vi "PCO_SetRecorderSubmode.vi"(8 "error in (no error)":errorcluster {"code" format="%x"}, 10 "wRecSubmode":u16(ring) items=["sequence", "ring buffer"], 11 "ph":u64) -> (0 "error out":errorcluster {"code" format="%x"}, 2 "ErrorMessage":i32 format="%x", 3 "ph out":u64)   [LabVIEW 2019, in "SDK.lvlib" / "RecordingControl.lvlib"]
doc: "<b>Description:</b>\nThis function sets the recorder submode of the camera. Recorder submode is only available if PCO_SetStorageMode is set to [recorder].\nRecorder submode can be set to [sequence] or [ring buffer].\n\n<b>-->RecorderSubmode: [sequence]</b>\nRecording is stopped, when the last buffer in the segment is reached\nNo images are overwritten\nRecording can be stopped by software\n\n<b>-->RecorderSubmode: [ring buffer]</b>\nCamera records continuously into ring buffer\nThe oldest images are overwritten, if a buffer overflows occures due to long recording times\nRecording must be stopped by software or with an stop event\n\n<b>Supported camera type:</b>\npco.dimax, pco.pixelfly usb, pco.ultraviolet, pco.1200, pco.1300, pco.1400, pco.1600, pco.2000, pco.4000\n\n<b>Descriptor dependency:</b>\ndwGeneralCapsDESC1: NO_RECORDER"
uses:
  RecordingControl.lvlib
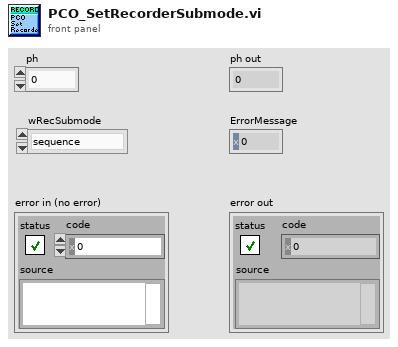
[diagram p1: front panel]
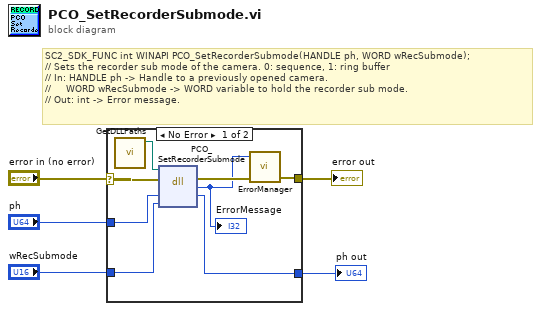
[diagram p0: block diagram]
diagram:
  # "SC2_SDK_FUNC int WINAPI PCO_SetRecorderSubmode(HANDLE ph, WORD wRecSubmode);\n// Sets the recorder sub mode of the camera. 0: sequence, 1: ring buffer\n// In: HANDLE ph -> Handle to a previously opened camera.\n//     WORD wRecSubmode -> WORD variable to hold the recorder sub mode.\n// Out: int -> Error message."
  n1 = case shown="No Error" "error in (no error)" {
    selector: "error in (no error)" -> [w10 w15]
    tunnel: "ph" -> [w13 w14]
    tunnel: [w12 w14] -> w4
    tunnel: "wRecSubmode" -> [w11 _]
    tunnel: [w8 w15] -> w2
    frame No Error {
      n2 = call "GetDLLPaths.vi"() -> ("SC2_Cam_Path"=w6:path)  [unwired: 9 in, 2 out]
      n3 = dll-call lib="?" fn="PCO_SetRecorderSubmode"(path in=w6, error in=w10, "ph"=w13, "wRecSubmode"=w11) -> (error out=w9:errorcluster, "return type"=w7:i32, "ph"=w12:u64)  [unwired: 2 in, 1 out]
      "ErrorMessage" <- w7
      n4 = call "ErrorManager.vi"("error in (no error)"=w9, "error code"=w7) -> ("error out"=w8:errorcluster)  [unwired: 3 in]
    }
    frame Error {
    }
  }
  "ph out" <- w4
  "error out" <- w2
